vi "_r2aio_16bit_8out_canopen_master.vi"() -> ()   [LabVIEW 2011]
panel:
  out "ret transmit_can_pdo 2":i16
  out "ret transmit_can_pdo 1":i16
  out "ret write_pdo_mapping 12":i16
  in  "Analogue OUT 8":i16
  out "ret write_node_object_dictionary 8":i16
  in  "Analogue OUT 7":i16
  out "ret write_node_object_dictionary 7":i16
  in  "Analogue OUT 6":i16
  out "ret write_node_object_dictionary 6":i16
  in  "Analogue OUT 5":i16
  out "ret write_node_object_dictionary 5":i16
  in  "Analogue OUT 4":i16
  out "ret write_node_object_dictionary 4":i16
  in  "Analogue OUT 3":i16
  out "ret write_node_object_dictionary 3":i16
  in  "Analogue OUT 2":i16
  out "ret write_node_object_dictionary 2":i16
  in  "Analogue OUT 1":i16
  out "ret write_pdo_mapping 11":i16
  out "ret write_pdo_mapping 10":i16
  out "ret write_pdo_mapping 9":i16
  out "ret write_pdo_mapping 8":i16
  out "ret write_pdo_mapping 7":i16
  out "ret write_pdo_mapping 6":i16
  out "ret write_pdo_mapping 5":i16
  out "ret write_pdo_mapping 4":i16
  out "ret write_pdo_mapping 2":i16
  out "ret add_node_object_dictionary 6411-8":i16
  out "ret add_node_object_dictionary 6411-7":i16
  out "ret add_node_object_dictionary 6411-6":i16
  out "ret add_node_object_dictionary 6411-5":i16
  out "ret add_node_object_dictionary 6411-4":i16
  out "ret add_node_object_dictionary 6411-3":i16
  out "ret add_node_object_dictionary 6411-2":i16
  out "datasize":u32
  out "Manufacturer software ver":string
  out "ret read_device_object_sdo 3":i16
  out "datasize":u32
  out "Manufacturer hardware ver":string
  out "ret read_device_object_sdo 2":i16
  out "datasize":u32
  out "Manufacturer dev name":string
  out "ret read_device_object_sdo 1":i16
  out "ret write_node_object_dictionary 1":i16
  in  "stop monitor":bool
  out "ret write_master_hbt":i16
  out "ret stop_can_master":i16
  out "ret write_pdo_mapping 3":i16
  out "ret write_pdo_mapping 1":i16
  out "ret add_node_object_dictionary 6411-1":i16
  out "ret write_device_object_sdo HBT":i16
  in  "slave node":u8
  in  "baudrate":T1(ring)
  in  "net":u8
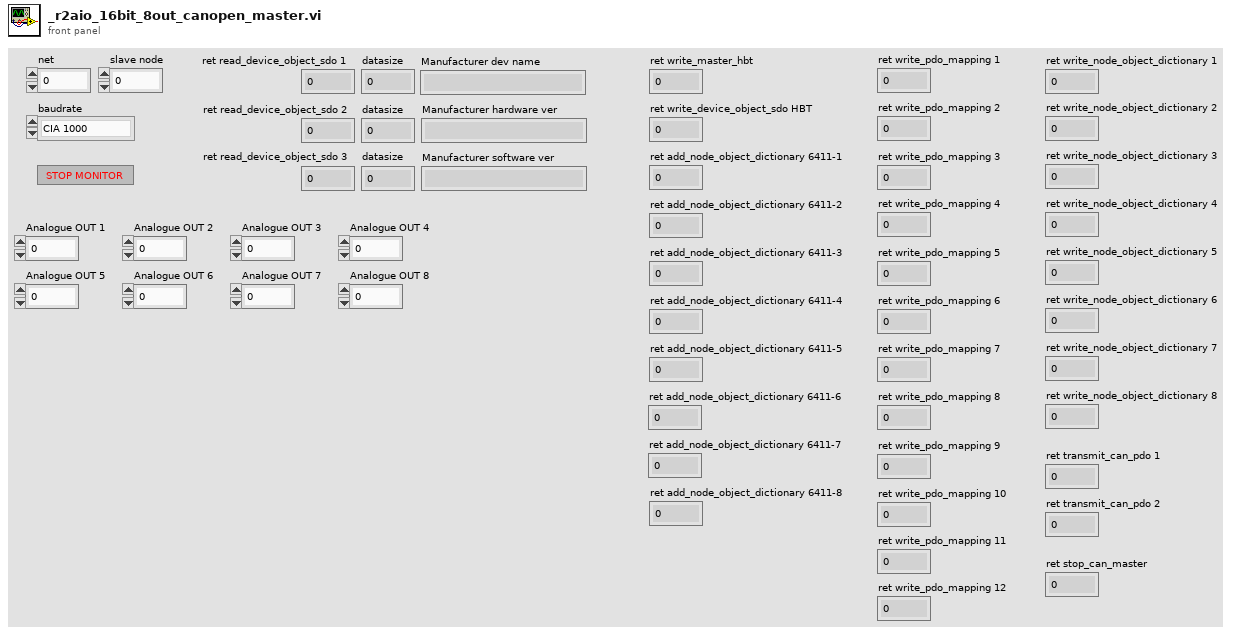
[diagram p1: front panel]
types:
  T1 = enum8{"CIA 1000", "CIA 800", "CIA 500", "CIA 250", "CIA 125", "CIA 100", "CIA 50", "CIA 20", "CIA 10", "CIA AUTO"}
diagram:
  n1 = flat-sequence {
    tunnel: ["slave node"] -> w51
    tunnel: w51 -> [w61]
    tunnel: [w61] -> w50
    tunnel: w50 -> [w63]
    tunnel: [w63] -> w53
    tunnel: w53 -> [w70]
    tunnel: [w70] -> w52
    tunnel: w52 -> [w73]
    tunnel: [w73] -> w48
    tunnel: w48 -> [w78]
    tunnel: [w78] -> w47
    tunnel: w47 -> [w83]
    tunnel: [w83] -> w46
    tunnel: w46 -> [w88]
    tunnel: [w88] -> w45
    tunnel: w45 -> [w93]
    tunnel: [w93] -> w44
    tunnel: w44 -> [w98]
    tunnel: [w98] -> w43
    tunnel: w43 -> [w104]
    tunnel: [w104] -> w42
    tunnel: w42 -> [w108]
    tunnel: [w108] -> w17
    tunnel: [w113] -> w49
    tunnel: w17 -> [w113]
    tunnel: [w118] -> w41
    tunnel: w49 -> [w118]
    tunnel: [w115] -> w29
    tunnel: w41 -> [w128]
    tunnel: [w128] -> w30
    tunnel: w29 -> [w126]
    tunnel: [w126] -> w28
    tunnel: [w135] -> w40
    tunnel: [w133] -> w27
    tunnel: w30 -> [w135]
    tunnel: w28 -> [w133]
    tunnel: w40 -> [w142]
    tunnel: [w142] -> w39
    tunnel: w27 -> [w140]
    tunnel: [w140] -> w26
    tunnel: w39 -> [w148]
    tunnel: [w148] -> w38
    tunnel: w26 -> [w147]
    tunnel: [w147] -> w25
    tunnel: w38 -> [w156]
    tunnel: [w156] -> w37
    tunnel: w25 -> [w154]
    tunnel: [w154] -> w24
    tunnel: w37 -> [w162]
    tunnel: [w162] -> w36
    tunnel: w24 -> [w161]
    tunnel: [w161] -> w23
    tunnel: w36 -> [w170]
    tunnel: [w170] -> w35
    tunnel: w23 -> [w168]
    tunnel: [w168] -> w22
    tunnel: w35 -> [w176]
    tunnel: [w176] -> w34
    tunnel: w22 -> [w175]
    tunnel: [w175] -> w21
    tunnel: w34 -> [w183]
    tunnel: [w183] -> w33
    tunnel: w21 -> [w182]
    tunnel: [w182] -> w20
    tunnel: [w191] -> w32
    tunnel: [w189] -> w19
    tunnel: w20 -> [w189]
    tunnel: w33 -> [w191]
    tunnel: w32 -> [w198]
    tunnel: [w198] -> w31
    tunnel: w19 -> [w196]
    tunnel: [w196] -> w18
    tunnel: [w205] -> w13
    tunnel: w31 -> [w205]
    tunnel: w18 -> [w203]
    tunnel: [w203] -> w1
    tunnel: [w214] -> w15
    tunnel: w13 -> [w214]
    tunnel: [w206] -> w2
    tunnel: w1 -> [w206]
    tunnel: w15 -> [w217]
    tunnel: [w217] -> w14
    tunnel: [w215] -> w3
    tunnel: w2 -> [w215]
    tunnel: w14 -> [w219]
    tunnel: [w219] -> w12
    tunnel: [w218] -> w4
    tunnel: w3 -> [w218]
    tunnel: w12 -> [w229]
    tunnel: [w229] -> w11
    tunnel: [w227] -> w5
    tunnel: w4 -> [w227]
    tunnel: w11 -> [w231]
    tunnel: [w231] -> w10
    tunnel: [w230] -> w6
    tunnel: w5 -> [w230]
    tunnel: w10 -> [w241]
    tunnel: [w241] -> w9
    tunnel: [w239] -> w7
    tunnel: w6 -> [w239]
    tunnel: w9 -> [w244]
    tunnel: [w244] -> w16
    tunnel: [w242] -> w8
    tunnel: w7 -> [w242]
    tunnel: w16 -> [w246]
    tunnel: w8 -> [w245]
    frame #0 {
      # "Start CAN master"
      n2 = call "start_can_master.vi"("br"="baudrate", "net"="net") -> ("return"=w57:i16)  [unwired: 9 in]
      n3 = Not Equal To 0?(x=w57) -> (x != 0?=w56:bool)
      n4 = Stop(stop? (T)=w56) -> ()
    }
    frame #1 {
      w59 = u8 129 items=["CAN_NMT_CS_DUMMY"=0, "CAN_NMT_START_REMOTE_NODE"=1, "CAN_NMT_STOP_REMOTE_NODE"=2, "CAN_NMT_ENTER_PRE_OPERATIONAL"=128, "CAN_NMT_RESET_NODE"=129, "CAN_NMT_RESET_COMMUNICATION"=130]  # NMT spec
      # "NMT Reset node"
      n5 = call "nmt_master_command.vi"("node"="slave node", "cs"=w59) -> ()  [unwired: 10 in]
    }
    frame #2 {
      n6 = Wait (ms)(milliseconds to wait=u32 500) -> ()  [unwired: 1 out]
    }
    frame #3 {
      # "Configure MASTER Heartbeat"
      n7 = call "write_master_hbt.vi"("hbt"=u16 1200, "node"=w63) -> ("return"=→"ret write_master_hbt":i16)  [unwired: 9 in]
    }
    frame #4 {
      # "Configure SLAVE Heartbeat"
      n8 = Build Array(u8 232, u8 3) -> (w66:u8[])
      n9 = call "write_device_object_sdo.vi"("node"=w70, "index"=u16 4119, "subind"=u8 0, "data"=w66, "datasize"=u32 2) -> ("return"=→"ret write_device_object_sdo HBT":i16)  [unwired: 10 in]
    }
    frame #5 {
      w75 = u16 3 items=["CAN_DEFTYPE_BOOLEAN"=1, "CAN_DEFTYPE_INTEGER8"=2, "CAN_DEFTYPE_INTEGER16"=3, "CAN_DEFTYPE_INTEGER32"=4, "CAN_DEFTYPE_UNSIGNED8"=5, "CAN_DEFTYPE_UNSIGNED16"=6, "CAN_DEFTYPE_UNSIGNED32"=7, "CAN_DEFTYPE_REAL32"=8, "CAN_DEFTYPE_VISIBLE_STRING"=9, "CAN_DEFTYPE_OCTET_STRING"=10, "CAN_DEFTYPE_UNICODE_STRING"=11, "CAN_DEFTYPE_TIME_OF_DAY"=12, "CAN_DEFTYPE_TIME_DIFFERENCE"=13, "CAN_DEFTYPE_DOMAIN"=15, "CAN_DEFTYPE_INTEGER24"=16, "CAN_DEFTYPE_REAL64"=17, "CAN_DEFTYPE_INTEGER40"=18, "CAN_DEFTYPE_INTEGER48"=19, "CAN_DEFTYPE_INTEGER56"=20, "CAN_DEFTYPE_INTEGER64"=21, "CAN_DEFTYPE_UNSIGNED24"=22, "CAN_DEFTYPE_UNSIGNED40"=24, "CAN_DEFTYPE_UNSIGNED48"=25, "CAN_DEFTYPE_UNSIGNED56"=26, "CAN_DEFTYPE_UNSIGNED64"=27]  # Data type spec
      # "Add Write Analogue output 1 object to MASTER dictionary"
      n10 = call "add_node_object_dictionary.vi"("type"=w75, "subind"=u8 1, "index"=u16 25617, "node"=w73) -> ("return"=→"ret add_node_object_dictionary 6411-1":i16)  [unwired: 7 in]
    }
    frame #6 {
      w80 = u16 3 items=["CAN_DEFTYPE_BOOLEAN"=1, "CAN_DEFTYPE_INTEGER8"=2, "CAN_DEFTYPE_INTEGER16"=3, "CAN_DEFTYPE_INTEGER32"=4, "CAN_DEFTYPE_UNSIGNED8"=5, "CAN_DEFTYPE_UNSIGNED16"=6, "CAN_DEFTYPE_UNSIGNED32"=7, "CAN_DEFTYPE_REAL32"=8, "CAN_DEFTYPE_VISIBLE_STRING"=9, "CAN_DEFTYPE_OCTET_STRING"=10, "CAN_DEFTYPE_UNICODE_STRING"=11, "CAN_DEFTYPE_TIME_OF_DAY"=12, "CAN_DEFTYPE_TIME_DIFFERENCE"=13, "CAN_DEFTYPE_DOMAIN"=15, "CAN_DEFTYPE_INTEGER24"=16, "CAN_DEFTYPE_REAL64"=17, "CAN_DEFTYPE_INTEGER40"=18, "CAN_DEFTYPE_INTEGER48"=19, "CAN_DEFTYPE_INTEGER56"=20, "CAN_DEFTYPE_INTEGER64"=21, "CAN_DEFTYPE_UNSIGNED24"=22, "CAN_DEFTYPE_UNSIGNED40"=24, "CAN_DEFTYPE_UNSIGNED48"=25, "CAN_DEFTYPE_UNSIGNED56"=26, "CAN_DEFTYPE_UNSIGNED64"=27]  # Data type spec
      # "Add Write Analogue output 2 object to MASTER dictionary"
      n11 = call "add_node_object_dictionary.vi"("type"=w80, "subind"=u8 2, "index"=u16 25617, "node"=w78) -> ("return"=→"ret add_node_object_dictionary 6411-2":i16)  [unwired: 7 in]
    }
    frame #7 {
      w85 = u16 3 items=["CAN_DEFTYPE_BOOLEAN"=1, "CAN_DEFTYPE_INTEGER8"=2, "CAN_DEFTYPE_INTEGER16"=3, "CAN_DEFTYPE_INTEGER32"=4, "CAN_DEFTYPE_UNSIGNED8"=5, "CAN_DEFTYPE_UNSIGNED16"=6, "CAN_DEFTYPE_UNSIGNED32"=7, "CAN_DEFTYPE_REAL32"=8, "CAN_DEFTYPE_VISIBLE_STRING"=9, "CAN_DEFTYPE_OCTET_STRING"=10, "CAN_DEFTYPE_UNICODE_STRING"=11, "CAN_DEFTYPE_TIME_OF_DAY"=12, "CAN_DEFTYPE_TIME_DIFFERENCE"=13, "CAN_DEFTYPE_DOMAIN"=15, "CAN_DEFTYPE_INTEGER24"=16, "CAN_DEFTYPE_REAL64"=17, "CAN_DEFTYPE_INTEGER40"=18, "CAN_DEFTYPE_INTEGER48"=19, "CAN_DEFTYPE_INTEGER56"=20, "CAN_DEFTYPE_INTEGER64"=21, "CAN_DEFTYPE_UNSIGNED24"=22, "CAN_DEFTYPE_UNSIGNED40"=24, "CAN_DEFTYPE_UNSIGNED48"=25, "CAN_DEFTYPE_UNSIGNED56"=26, "CAN_DEFTYPE_UNSIGNED64"=27]  # Data type spec
      # "Add Write Analogue output 3 object to MASTER dictionary"
      n12 = call "add_node_object_dictionary.vi"("type"=w85, "subind"=u8 3, "index"=u16 25617, "node"=w83) -> ("return"=→"ret add_node_object_dictionary 6411-3":i16)  [unwired: 7 in]
    }
    frame #8 {
      w90 = u16 3 items=["CAN_DEFTYPE_BOOLEAN"=1, "CAN_DEFTYPE_INTEGER8"=2, "CAN_DEFTYPE_INTEGER16"=3, "CAN_DEFTYPE_INTEGER32"=4, "CAN_DEFTYPE_UNSIGNED8"=5, "CAN_DEFTYPE_UNSIGNED16"=6, "CAN_DEFTYPE_UNSIGNED32"=7, "CAN_DEFTYPE_REAL32"=8, "CAN_DEFTYPE_VISIBLE_STRING"=9, "CAN_DEFTYPE_OCTET_STRING"=10, "CAN_DEFTYPE_UNICODE_STRING"=11, "CAN_DEFTYPE_TIME_OF_DAY"=12, "CAN_DEFTYPE_TIME_DIFFERENCE"=13, "CAN_DEFTYPE_DOMAIN"=15, "CAN_DEFTYPE_INTEGER24"=16, "CAN_DEFTYPE_REAL64"=17, "CAN_DEFTYPE_INTEGER40"=18, "CAN_DEFTYPE_INTEGER48"=19, "CAN_DEFTYPE_INTEGER56"=20, "CAN_DEFTYPE_INTEGER64"=21, "CAN_DEFTYPE_UNSIGNED24"=22, "CAN_DEFTYPE_UNSIGNED40"=24, "CAN_DEFTYPE_UNSIGNED48"=25, "CAN_DEFTYPE_UNSIGNED56"=26, "CAN_DEFTYPE_UNSIGNED64"=27]  # Data type spec
      # "Add Write Analogue output 4 object to MASTER dictionary"
      n13 = call "add_node_object_dictionary.vi"("type"=w90, "subind"=u8 4, "index"=u16 25617, "node"=w88) -> ("return"=→"ret add_node_object_dictionary 6411-4":i16)  [unwired: 7 in]
    }
    frame #9 {
      w95 = u16 3 items=["CAN_DEFTYPE_BOOLEAN"=1, "CAN_DEFTYPE_INTEGER8"=2, "CAN_DEFTYPE_INTEGER16"=3, "CAN_DEFTYPE_INTEGER32"=4, "CAN_DEFTYPE_UNSIGNED8"=5, "CAN_DEFTYPE_UNSIGNED16"=6, "CAN_DEFTYPE_UNSIGNED32"=7, "CAN_DEFTYPE_REAL32"=8, "CAN_DEFTYPE_VISIBLE_STRING"=9, "CAN_DEFTYPE_OCTET_STRING"=10, "CAN_DEFTYPE_UNICODE_STRING"=11, "CAN_DEFTYPE_TIME_OF_DAY"=12, "CAN_DEFTYPE_TIME_DIFFERENCE"=13, "CAN_DEFTYPE_DOMAIN"=15, "CAN_DEFTYPE_INTEGER24"=16, "CAN_DEFTYPE_REAL64"=17, "CAN_DEFTYPE_INTEGER40"=18, "CAN_DEFTYPE_INTEGER48"=19, "CAN_DEFTYPE_INTEGER56"=20, "CAN_DEFTYPE_INTEGER64"=21, "CAN_DEFTYPE_UNSIGNED24"=22, "CAN_DEFTYPE_UNSIGNED40"=24, "CAN_DEFTYPE_UNSIGNED48"=25, "CAN_DEFTYPE_UNSIGNED56"=26, "CAN_DEFTYPE_UNSIGNED64"=27]  # Data type spec
      # "Add Write Analogue output 5 object to MASTER dictionary"
      n14 = call "add_node_object_dictionary.vi"("type"=w95, "subind"=u8 5, "index"=u16 25617, "node"=w93) -> ("return"=→"ret add_node_object_dictionary 6411-5":i16)  [unwired: 7 in]
    }
    frame #10 {
      w100 = u16 3 items=["CAN_DEFTYPE_BOOLEAN"=1, "CAN_DEFTYPE_INTEGER8"=2, "CAN_DEFTYPE_INTEGER16"=3, "CAN_DEFTYPE_INTEGER32"=4, "CAN_DEFTYPE_UNSIGNED8"=5, "CAN_DEFTYPE_UNSIGNED16"=6, "CAN_DEFTYPE_UNSIGNED32"=7, "CAN_DEFTYPE_REAL32"=8, "CAN_DEFTYPE_VISIBLE_STRING"=9, "CAN_DEFTYPE_OCTET_STRING"=10, "CAN_DEFTYPE_UNICODE_STRING"=11, "CAN_DEFTYPE_TIME_OF_DAY"=12, "CAN_DEFTYPE_TIME_DIFFERENCE"=13, "CAN_DEFTYPE_DOMAIN"=15, "CAN_DEFTYPE_INTEGER24"=16, "CAN_DEFTYPE_REAL64"=17, "CAN_DEFTYPE_INTEGER40"=18, "CAN_DEFTYPE_INTEGER48"=19, "CAN_DEFTYPE_INTEGER56"=20, "CAN_DEFTYPE_INTEGER64"=21, "CAN_DEFTYPE_UNSIGNED24"=22, "CAN_DEFTYPE_UNSIGNED40"=24, "CAN_DEFTYPE_UNSIGNED48"=25, "CAN_DEFTYPE_UNSIGNED56"=26, "CAN_DEFTYPE_UNSIGNED64"=27]  # Data type spec
      # "Add Write Analogue output 6 object to MASTER dictionary"
      n15 = call "add_node_object_dictionary.vi"("type"=w100, "subind"=u8 6, "index"=u16 25617, "node"=w98) -> ("return"=→"ret add_node_object_dictionary 6411-6":i16)  [unwired: 7 in]
    }
    frame #11 {
      w103 = u16 3 items=["CAN_DEFTYPE_BOOLEAN"=1, "CAN_DEFTYPE_INTEGER8"=2, "CAN_DEFTYPE_INTEGER16"=3, "CAN_DEFTYPE_INTEGER32"=4, "CAN_DEFTYPE_UNSIGNED8"=5, "CAN_DEFTYPE_UNSIGNED16"=6, "CAN_DEFTYPE_UNSIGNED32"=7, "CAN_DEFTYPE_REAL32"=8, "CAN_DEFTYPE_VISIBLE_STRING"=9, "CAN_DEFTYPE_OCTET_STRING"=10, "CAN_DEFTYPE_UNICODE_STRING"=11, "CAN_DEFTYPE_TIME_OF_DAY"=12, "CAN_DEFTYPE_TIME_DIFFERENCE"=13, "CAN_DEFTYPE_DOMAIN"=15, "CAN_DEFTYPE_INTEGER24"=16, "CAN_DEFTYPE_REAL64"=17, "CAN_DEFTYPE_INTEGER40"=18, "CAN_DEFTYPE_INTEGER48"=19, "CAN_DEFTYPE_INTEGER56"=20, "CAN_DEFTYPE_INTEGER64"=21, "CAN_DEFTYPE_UNSIGNED24"=22, "CAN_DEFTYPE_UNSIGNED40"=24, "CAN_DEFTYPE_UNSIGNED48"=25, "CAN_DEFTYPE_UNSIGNED56"=26, "CAN_DEFTYPE_UNSIGNED64"=27]  # Data type spec
      # "Add Write Analogue output 7 object to MASTER dictionary"
      n16 = call "add_node_object_dictionary.vi"("type"=w103, "subind"=u8 7, "index"=u16 25617, "node"=w104) -> ("return"=→"ret add_node_object_dictionary 6411-7":i16)  [unwired: 7 in]
    }
    frame #12 {
      w110 = u16 3 items=["CAN_DEFTYPE_BOOLEAN"=1, "CAN_DEFTYPE_INTEGER8"=2, "CAN_DEFTYPE_INTEGER16"=3, "CAN_DEFTYPE_INTEGER32"=4, "CAN_DEFTYPE_UNSIGNED8"=5, "CAN_DEFTYPE_UNSIGNED16"=6, "CAN_DEFTYPE_UNSIGNED32"=7, "CAN_DEFTYPE_REAL32"=8, "CAN_DEFTYPE_VISIBLE_STRING"=9, "CAN_DEFTYPE_OCTET_STRING"=10, "CAN_DEFTYPE_UNICODE_STRING"=11, "CAN_DEFTYPE_TIME_OF_DAY"=12, "CAN_DEFTYPE_TIME_DIFFERENCE"=13, "CAN_DEFTYPE_DOMAIN"=15, "CAN_DEFTYPE_INTEGER24"=16, "CAN_DEFTYPE_REAL64"=17, "CAN_DEFTYPE_INTEGER40"=18, "CAN_DEFTYPE_INTEGER48"=19, "CAN_DEFTYPE_INTEGER56"=20, "CAN_DEFTYPE_INTEGER64"=21, "CAN_DEFTYPE_UNSIGNED24"=22, "CAN_DEFTYPE_UNSIGNED40"=24, "CAN_DEFTYPE_UNSIGNED48"=25, "CAN_DEFTYPE_UNSIGNED56"=26, "CAN_DEFTYPE_UNSIGNED64"=27]  # Data type spec
      # "Add Write Analogue output 8 object to MASTER dictionary"
      n17 = call "add_node_object_dictionary.vi"("type"=w110, "subind"=u8 8, "index"=u16 25617, "node"=w108) -> ("return"=→"ret add_node_object_dictionary 6411-8":i16)  [unwired: 7 in]
    }
    frame #13 {
      w114 = u8 1 items=["CAN_NMT_CS_DUMMY"=0, "CAN_NMT_START_REMOTE_NODE"=1, "CAN_NMT_STOP_REMOTE_NODE"=2, "CAN_NMT_ENTER_PRE_OPERATIONAL"=128, "CAN_NMT_RESET_NODE"=129, "CAN_NMT_RESET_COMMUNICATION"=130]  # NMT spec
      # "NMT Start remote node"
      n18 = call "nmt_master_command.vi"("node"=w113, "cs"=w114) -> ()  [unwired: 10 in]
    }
    frame #14 {
      # "Disable TPDO2 mapping"
      n19 = Subtract(x=w118, y=u8 1) -> (x-y=w117:u8)
      n20 = Multiply(x=w117, y=u8 4) -> (x*y=w116:u8)
      n21 = To Unsigned Word Integer(number=w116) -> (unsigned 16bit integer=w115:u16)
      n22 = Add(x=w115, y=u16 6657) -> (x+y=w121:u16)
      n23 = call "write_pdo_mapping.vi"("data"=u32 0, "subind"=u8 0, "index"=w121) -> ("return"=→"ret write_pdo_mapping 1":i16)  [unwired: 8 in]
    }
    frame #15 {
      # "Disable TPDO3 mapping"
      n24 = Add(x=w126, y=u16 6658) -> (x+y=w127:u16)
      n25 = call "write_pdo_mapping.vi"("data"=u32 0, "subind"=u8 0, "index"=w127) -> ("return"=→"ret write_pdo_mapping 2":i16)  [unwired: 8 in]
    }
    frame #16 {
      # "Map Write Analogue Output 1 TPDO2"
      n26 = Add(x=w133, y=u16 6657) -> (x+y=w134:u16)
      n27 = call "write_pdo_mapping.vi"("data"=u32 1678835984, "subind"=u8 1, "index"=w134) -> ("return"=→"ret write_pdo_mapping 3":i16)  [unwired: 8 in]
    }
    frame #17 {
      # "Map Write Analogue Output 2 TPDO2"
      n28 = Add(x=w140, y=u16 6657) -> (x+y=w141:u16)
      n29 = call "write_pdo_mapping.vi"("data"=u32 1678836240, "subind"=u8 2, "index"=w141) -> ("return"=→"ret write_pdo_mapping 4":i16)  [unwired: 8 in]
    }
    frame #18 {
      # "Map Write Analogue Output 3 TPDO2"
      n30 = Add(x=w147, y=u16 6657) -> (x+y=w150:u16)
      n31 = call "write_pdo_mapping.vi"("data"=u32 1678836496, "subind"=u8 3, "index"=w150) -> ("return"=→"ret write_pdo_mapping 5":i16)  [unwired: 8 in]
    }
    frame #19 {
      # "Map Write Analogue Output 4 TPDO2"
      n32 = Add(x=w154, y=u16 6657) -> (x+y=w155:u16)
      n33 = call "write_pdo_mapping.vi"("data"=u32 1678836752, "subind"=u8 4, "index"=w155) -> ("return"=→"ret write_pdo_mapping 6":i16)  [unwired: 8 in]
    }
    frame #20 {
      # "Map Write Analogue Output 5 TPDO3"
      n34 = Add(x=w161, y=u16 6658) -> (x+y=w163:u16)
      n35 = call "write_pdo_mapping.vi"("data"=u32 1678837008, "subind"=u8 1, "index"=w163) -> ("return"=→"ret write_pdo_mapping 7":i16)  [unwired: 8 in]
    }
    frame #21 {
      # "Map Write Analogue Output 6 TPDO3"
      n36 = Add(x=w168, y=u16 6658) -> (x+y=w169:u16)
      n37 = call "write_pdo_mapping.vi"("data"=u32 1678837264, "subind"=u8 2, "index"=w169) -> ("return"=→"ret write_pdo_mapping 8":i16)  [unwired: 8 in]
    }
    frame #22 {
      # "Map Write Analogue Output 7 TPDO3"
      n38 = Add(x=w175, y=u16 6658) -> (x+y=w178:u16)
      n39 = call "write_pdo_mapping.vi"("data"=u32 1678837520, "subind"=u8 3, "index"=w178) -> ("return"=→"ret write_pdo_mapping 9":i16)  [unwired: 8 in]
    }
    frame #23 {
      # "Map Write Analogue Output 8 TPDO3"
      n40 = Add(x=w182, y=u16 6658) -> (x+y=w185:u16)
      n41 = call "write_pdo_mapping.vi"("data"=u32 1678837776, "subind"=u8 4, "index"=w185) -> ("return"=→"ret write_pdo_mapping 10":i16)  [unwired: 8 in]
    }
    frame #24 {
      # "Enable TPDO2 mapping"
      n42 = Add(x=w189, y=u16 6657) -> (x+y=w190:u16)
      n43 = call "write_pdo_mapping.vi"("data"=u32 4, "subind"=u8 0, "index"=w190) -> ("return"=→"ret write_pdo_mapping 11":i16)  [unwired: 8 in]
    }
    frame #25 {
      # "Enable TPDO3 mapping"
      n44 = Add(x=w196, y=u16 6658) -> (x+y=w197:u16)
      n45 = call "write_pdo_mapping.vi"("data"=u32 4, "subind"=u8 0, "index"=w197) -> ("return"=→"ret write_pdo_mapping 12":i16)  [unwired: 8 in]
    }
    frame #26 {
      n46 = Wait (ms)(milliseconds to wait=u32 500) -> ()  [unwired: 1 out]
    }
    frame #27 {
      # "Read Manufacturer Device Name"
      n47 = call "read_device_object_sdo.vi"("node"=w214, "index"=u16 4104, "subind"=u8 0, "datasize"=u32 128) -> ("return"=→"ret read_device_object_sdo 1":i16, "data"=w209:u8[], "datasize"=→"datasize":u32)  [unwired: 9 in]
      n48 = Byte Array To String(unsigned byte array=w209) -> (string=→"Manufacturer dev name":string)
    }
    frame #28 {
      n49 = Wait (ms)(milliseconds to wait=u32 500) -> ()  [unwired: 1 out]
    }
    frame #29 {
      # "Read Manufacturer Hardware Version"
      n50 = call "read_device_object_sdo.vi"("node"=w219, "index"=u16 4105, "subind"=u8 0, "datasize"=u32 128) -> ("return"=→"ret read_device_object_sdo 2":i16, "data"=w222:u8[], "datasize"=→"datasize":u32)  [unwired: 9 in]
      n51 = Byte Array To String(unsigned byte array=w222) -> (string=→"Manufacturer hardware ver":string)
    }
    frame #30 {
      n52 = Wait (ms)(milliseconds to wait=u32 500) -> ()  [unwired: 1 out]
    }
    frame #31 {
      # "Read Manufacturer Software Version"
      n53 = call "read_device_object_sdo.vi"("node"=w231, "index"=u16 4106, "subind"=u8 0, "datasize"=u32 128) -> ("return"=→"ret read_device_object_sdo 3":i16, "data"=w234:u8[], "datasize"=→"datasize":u32)  [unwired: 9 in]
      n54 = Byte Array To String(unsigned byte array=w234) -> (string=→"Manufacturer software ver":string)
    }
    frame #32 {
      n55 = Wait (ms)(milliseconds to wait=u32 500) -> ()  [unwired: 1 out]
    }
    frame #33 {
      w243 = u8 1 items=["NOT_VALID", "VALID"]  # State
      # "Set all PDOs valid"
      n56 = call "set_all_pdos_state.vi"("state"=w243) -> ()  [unwired: 11 in]
    }
    frame #34 {
      # "Monitor"
      n57 = while {
        tunnel: w246 -> [w285]
        tunnel: w245 -> [w284]
        tunnel: w245 -> [w283]
        shift-right: ["Analogue OUT 8"] -> _
        shift-left: _ -> [w272]
        shift-left: _ -> [w273]
        shift-right: ["Analogue OUT 7"] -> _
        shift-left: _ -> [w270]
        shift-right: ["Analogue OUT 6"] -> _
        shift-left: _ -> [w268]
        shift-right: ["Analogue OUT 5"] -> _
        shift-left: _ -> [w260]
        shift-right: ["Analogue OUT 4"] -> _
        shift-left: _ -> [w266]
        shift-right: ["Analogue OUT 3"] -> _
        shift-left: _ -> [w264]
        shift-right: ["Analogue OUT 2"] -> _
        shift-left: _ -> [w262]
        shift-right: ["Analogue OUT 1"] -> _
        shift-left: _ -> [w258]
        shift-left: _ -> [w271]
        shift-left: _ -> [w269]
        shift-left: _ -> [w261]
        shift-left: _ -> [w267]
        shift-left: _ -> [w265]
        shift-left: _ -> [w263]
        shift-left: _ -> [w259]
        stop <- "stop monitor" stop-if-true
        n58 = Equal?(x=w272, y=w273) -> (x = y?=w274:bool)
        n59 = Equal?(x=w270, y=w271) -> (x = y?=w257:bool)
        n60 = Equal?(x=w268, y=w269) -> (x = y?=w256:bool)
        n61 = Equal?(x=w260, y=w261) -> (x = y?=w255:bool)
        n62 = Equal?(x=w266, y=w267) -> (x = y?=w254:bool)
        n63 = Equal?(x=w264, y=w265) -> (x = y?=w253:bool)
        n64 = Equal?(x=w262, y=w263) -> (x = y?=w252:bool)
        n65 = Equal?(x=w258, y=w259) -> (x = y?=w251:bool)
        n66 = To Unsigned Quad Integer(1:"Analogue OUT 1") -> (0:w317:u64)
        n67 = Build Array(w254, w253, w252, w251) -> (w249:bool[])
        n68 = Build Array(w274, w257, w256, w255) -> (w247:bool[])
        n69 = call "write_node_object_dictionary.vi"("num"=w317, "subind"=u8 1, "index"=u16 25617, "node"=w285) -> ("return"=→"ret write_node_object_dictionary 1":i16)  [unwired: 6 in, 1 out]
        n70 = And Array Elements(Boolean array=w249) -> (logical AND=w250:bool)
        n71 = case shown="False" w250 {
          tunnel: w284 -> [w323 _]
          frame False {
            n72 = Add(x=u16 6145, y=w323) -> (x+y=w325:u16)
            n73 = call "transmit_can_pdo.vi"("index"=w325) -> ("return"=→"ret transmit_can_pdo 1":i16)  [unwired: 10 in]
          }
          frame True {
          }
        }
        n74 = To Unsigned Quad Integer(1:"Analogue OUT 2") -> (0:w311:u64)
        n75 = call "write_node_object_dictionary.vi"("num"=w311, "subind"=u8 2, "index"=u16 25617, "node"=w285) -> ("return"=→"ret write_node_object_dictionary 2":i16)  [unwired: 6 in, 1 out]
        n76 = To Unsigned Quad Integer(1:"Analogue OUT 3") -> (0:w309:u64)
        n77 = call "write_node_object_dictionary.vi"("num"=w309, "subind"=u8 3, "index"=u16 25617, "node"=w285) -> ("return"=→"ret write_node_object_dictionary 3":i16)  [unwired: 6 in, 1 out]
        n78 = To Unsigned Quad Integer(1:"Analogue OUT 4") -> (0:w305:u64)
        n79 = call "write_node_object_dictionary.vi"("num"=w305, "subind"=u8 4, "index"=u16 25617, "node"=w285) -> ("return"=→"ret write_node_object_dictionary 4":i16)  [unwired: 6 in, 1 out]
        n80 = And Array Elements(Boolean array=w247) -> (logical AND=w248:bool)
        n81 = case shown="False" w248 {
          tunnel: w283 -> [w319 _]
          frame False {
            n82 = Add(x=u16 6146, y=w319) -> (x+y=w322:u16)
            n83 = call "transmit_can_pdo.vi"("index"=w322) -> ("return"=→"ret transmit_can_pdo 2":i16)  [unwired: 10 in]
          }
          frame True {
          }
        }
        n84 = To Unsigned Quad Integer(1:"Analogue OUT 5") -> (0:w301:u64)
        n85 = call "write_node_object_dictionary.vi"("num"=w301, "subind"=u8 5, "index"=u16 25617, "node"=w285) -> ("return"=→"ret write_node_object_dictionary 5":i16)  [unwired: 6 in, 1 out]
        n86 = To Unsigned Quad Integer(1:"Analogue OUT 6") -> (0:w297:u64)
        n87 = call "write_node_object_dictionary.vi"("num"=w297, "subind"=u8 6, "index"=u16 25617, "node"=w285) -> ("return"=→"ret write_node_object_dictionary 6":i16)  [unwired: 6 in, 1 out]
        n88 = To Unsigned Quad Integer(1:"Analogue OUT 7") -> (0:w294:u64)
        n89 = call "write_node_object_dictionary.vi"("num"=w294, "subind"=u8 7, "index"=u16 25617, "node"=w285) -> ("return"=→"ret write_node_object_dictionary 7":i16)  [unwired: 6 in, 1 out]
        n90 = To Unsigned Quad Integer(1:"Analogue OUT 8") -> (0:w289:u64)
        n91 = call "write_node_object_dictionary.vi"("num"=w289, "subind"=u8 8, "index"=u16 25617, "node"=w285) -> ("return"=→"ret write_node_object_dictionary 8":i16)  [unwired: 6 in, 1 out]
      }
    }
    frame #35 {
      # "Stop CAN master"
      n92 = call "stop_can_master.vi"() -> ("return"=→"ret stop_can_master":i16)  [unwired: 11 in]
    }
  }
